vi "niFpgaDcRmsInsideSCTLWindow.vi"(0 "input data":fxp<+/-,32,1>, 1 "reset":bool, 9 "input valid":bool, 12 "ready for output":bool=TRUE) -> (2 "Sum result":fxp<+/-,42,11> format="%.35g", 4 "DC result":fxp<+/-,32,1> format="%.32g", 6 "RMS result":fxp<+,32,1> format="%.32g", 8 "Mean Square result":fxp<+,63,1> format="%.63g", 10 "results valid":bool, 14 "ready for input":bool)   [LabVIEW 2017]
uses:
  <vilib>/rvi/FXPMathLib/basic elements/FxpIntAccumulator/subVIs/nifxpmath_IntAccumulator_SimConfig.ctl
  <vilib>/rvi/FXPMathLib/basic elements/FxpIntAccumulator/simVIs/DllFxpIntAccumulator_sub.vi
  <vilib>/rvi/FXPMathLib/basic elements/FxpIntAccumulator/XNode/nifxpmath_IntAccumulator.xnode
  <vilib>/fxp/LVFixedPointOverflowPolicyTypeDef.ctl
  <vilib>/rvi/FXPMathLib/FxpMul/XNode/nifxpmath_Multiplier.xnode
  <vilib>/rvi/FXPMathLib/FxpSqrt/XNode/nifxpmath_Sqrt.xnode
  <vilib>/rvi/FXPMathLib/FxpSqrt/simVIs/DllSqrtTemp_sub.vi
  <vilib>/rvi/FXPMathLib/FxpSqrt/subVIs/nifxpmath_Sqrt_SimConfig.ctl
  <vilib>/rvi/FXPMathLib/sim/FxpSim.dll
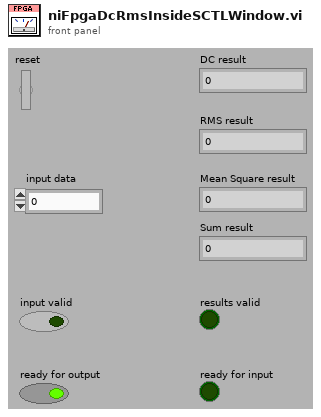
[diagram p1: front panel]
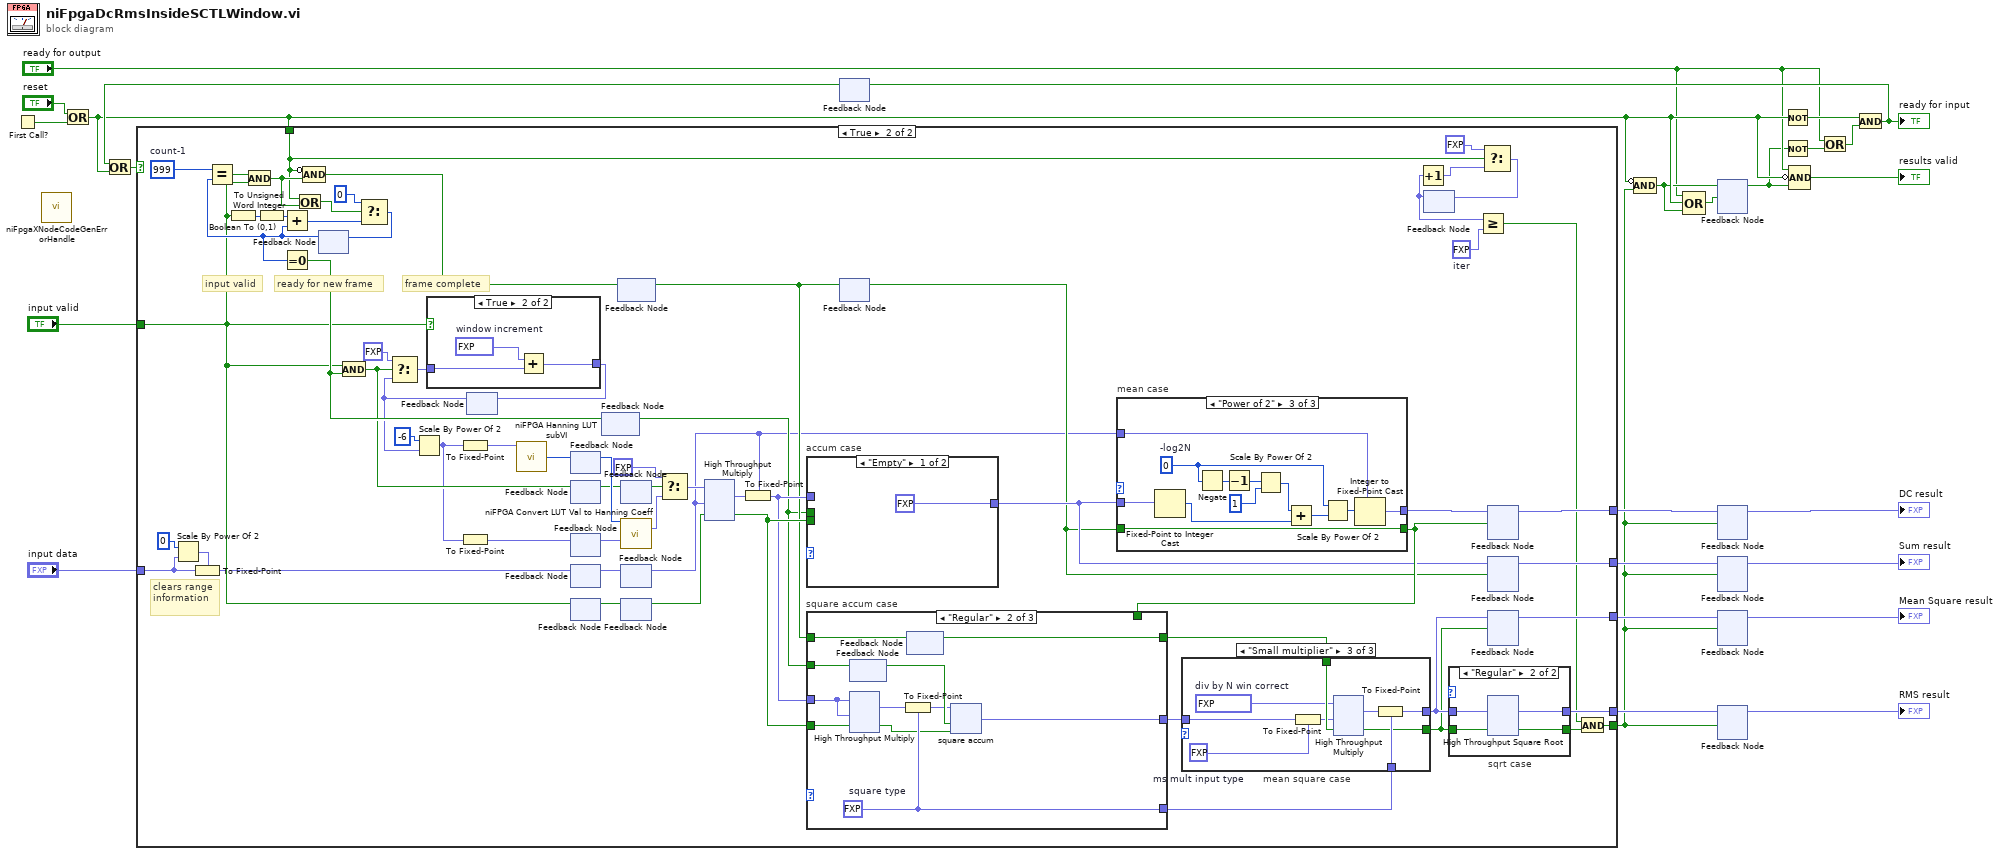
[diagram p0: block diagram]
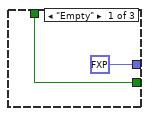
[diagram p4: hidden frame]
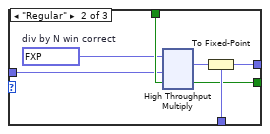
[diagram p5: hidden frame]
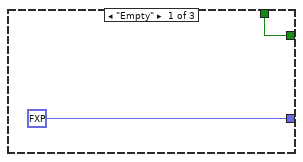
[diagram p6: hidden frame]
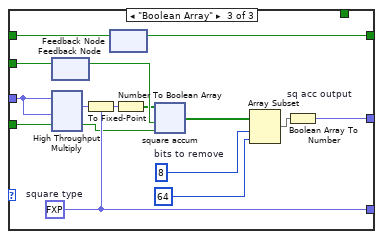
[diagram p7: hidden frame]
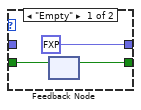
[diagram p8: hidden frame]
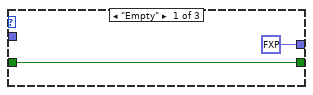
[diagram p9: hidden frame]
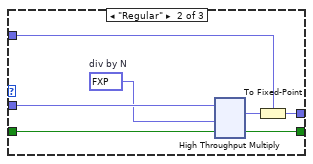
[diagram p10: hidden frame]
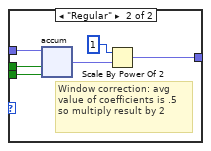
[diagram p11: hidden frame]
diagram:
  n1 = First Call?() -> (First Call?: T/F=w23:bool)
  n2 = call <vilib>:"niFpgaXNodeCodeGenErrorHandle.vi"() -> ()  [unwired: 1 in]
  n3 = Or(x="reset", y=w23) -> (x .or. y?=w6:bool)
  n4 = feedback #1() -> (w7:bool)  [unwired: 1 in]
  n5 = Or(x=w7, y=w6) -> (x .or. y?=w8:bool)
  n6 = case shown="True" w8 {
    tunnel: w6 -> [_ w78]
    tunnel: [_ w72] -> w16
    tunnel: [_ w71] -> w15
    tunnel: [_ w68] -> w14
    tunnel: [_ w66] -> w13
    tunnel: "input data" -> [_ w27]
    tunnel: "input valid" -> [_ w60]
    tunnel: [_ w52] -> w10
    frame False {
    }
    frame True {
      w80 = fxp<+,6,6> 43.0  # iter
      w76 = u16 999  # count-1
      # "clears range information"
      # "frame complete"
      # "ready for new frame"
      # "input valid"
      n7 = Scale By Power Of 2(n=0, x=w27) -> (x*2^n=w26:fxp<+/-,32,1>)
      n8 = To Fixed-Point(fixed-point type=w26, number=w27) -> (fixed-point=w42:fxp<+/-,32,1>)
      n9 = Boolean To (0,1)(Boolean=w60) -> (0, 1=w90:i16)
      n10 = To Unsigned Word Integer(number=w90) -> (unsigned 16bit integer=w75:u16)
      n11 = feedback #2() -> (w86:u16)  [unwired: 1 in]
      n12 = Equal?(x=w76, y=w86) -> (x = y?=w88:bool)
      n13 = And(x=w88, y=w60) -> (x .and. y?=w84:bool)
      n14 = Add(x=w75, y=w86) -> (x+y=w89:u16)
      n15 = Equal To 0?(x=w86) -> (x = 0?=w61:bool)
      n16 = Or(x=w78, y=w84) -> (x .or. y?=w85:bool)
      n17 = Compound Arithmetic op=AND(invert w78, w84) -> (w51:bool)
      n18 = And(x=w60, y=w61) -> (x .and. y?=w43:bool)
      n19 = Select(t=u16 0, s=w85, f=w89) -> (s? t:f=w77:u16)
      n20 = feedback-in #2(w77) -> ()
      n21 = feedback #3() -> (w39:fxp<+,32,16>)  [unwired: 1 in]
      n22 = Select(t=fxp<+,32,16> 0.0, s=w43, f=w39) -> (s? t:f=w62:fxp<+,32,16>)
      n23 = Scale By Power Of 2(n=-6, x=w39) -> (x*2^n=w38:fxp<+,32,16>)
      n24 = case shown="True" w60 {
        tunnel: [w91 w94] -> w63
        tunnel: w62 -> [w91 w92]
        frame False {
        }
        frame True {
          w93 = fxp<+,32,16> 65.53599548339844  # window increment
          n25 = Add(x=w93, y=w92) -> (x+y=w94:fxp<+,32,16>)
        }
      }
      n26 = To Fixed-Point(number=w38) -> (fixed-point=w30:fxp<+,10,10>)  [unwired: 1 in]
      n27 = To Fixed-Point(number=w38) -> (fixed-point=w40:fxp<+,16,0>)  [unwired: 1 in]
      n28 = feedback-in #3(w63) -> ()
      n29 = call <vilib>:"niFPGA Hanning LUT subVI.vi"("address"=w30) -> ("data out"=w29:u32)  [unwired: 7 in]
      n30 = feedback-in #4(w29) -> ()
      n31 = feedback #4() -> (w55:u32)  [unwired: 1 in]
      n32 = feedback-in #5(w43) -> ()
      n33 = feedback #5() -> (w32:bool)  [unwired: 1 in]
      n34 = feedback-in #6(w40) -> ()
      n35 = feedback #6() -> (w54:fxp<+,16,0>)  [unwired: 1 in]
      n36 = feedback-in #7(w42) -> ()
      n37 = feedback #7() -> (w36:fxp<+/-,32,1>)  [unwired: 1 in]
      n38 = feedback-in #8(w60) -> ()
      n39 = feedback #8() -> (w35:bool)  [unwired: 1 in]
      n40 = feedback-in #9(w61) -> ()
      n41 = feedback #9() -> (w48:bool)  [unwired: 1 in]
      n42 = feedback-in #10(w51) -> ()
      n43 = feedback #10() -> (w50:bool)  [unwired: 1 in]
      n44 = feedback-in #11(w32) -> ()
      n45 = feedback #11() -> (w31:bool)  [unwired: 1 in]
      n46 = call <vilib>:"niFPGA Convert LUT Val to Hanning Coeff.vi"("LUT value"=w55, "fractional index"=w54) -> ("Hanning coefficient"=w46:fxp<+,17,0>)  [unwired: 13 in]
      n47 = feedback-in #12(w36) -> ()
      n48 = feedback #12() -> (w33:fxp<+/-,32,1>)  [unwired: 1 in]
      n49 = feedback-in #13(w35) -> ()
      n50 = feedback #13() -> (w34:bool)  [unwired: 1 in]
      n51 = Select(t=fxp<+,17,0> 0.0, s=w31, f=w46) -> (s? t:f=w45:fxp<+,17,0>)
      n52 = xnode "High Throughput Multiply"("x"=w45, "y"=w33, "input valid"=w34) -> ("x*y"=w57:fxp<+/-,49,1>, "output valid"=w59:bool)  [unwired: 1 in, 1 out]
      n53 = To Fixed-Point(fixed-point type=w33, number=w57) -> (fixed-point=w56:fxp<+/-,32,1>)
      n54 = case "accum case" shown="\"Empty\"" {
        selector: _ -> [_ _]
        tunnel: w59 -> [_ w249]
        tunnel: w48 -> [_ w248]
        tunnel: w56 -> [_ w247]
        tunnel: [fxp<+/-,26,11> 0.0 ("s") w244] -> w58
        frame "Empty" {
        }
        frame "Regular" {
          # "Window correction: avg value of coefficients is .5 so multiply result by 2"
          n55 = xnode "accum"("x"=w247, "load (F)"=w248, "enable (T)"=w249) -> ("s"=w245:fxp<+/-,48,17>)  [unwired: 2 in, 1 out]
          n56 = Scale By Power Of 2(n=1, x=w245) -> (x*2^n=w244:fxp<+/-,48,17>)
        }
      }
      n57 = feedback-in #14(w50) -> ()
      n58 = feedback #14() -> (w49:bool)  [unwired: 1 in]
      n59 = case "mean case" shown="\"Power of 2\"" {
        selector: _ -> [_ _ _]
        tunnel: w33 -> [_ w230 w234]
        tunnel: w49 -> [w223 w229 w242]
        tunnel: w58 -> [_ w228 w232]
        tunnel: [w223 w227 w242] -> w65
        tunnel: [fxp<+/-,16,1> 0.0 ("input data") w226 w231] -> w67
        frame "Empty" {
        }
        frame "Regular" {
          w224 = fxp<+,17,-9> 0.0010000020265579224  # div by N
          n60 = xnode "High Throughput Multiply"("x"=w228, "y"=w224, "input valid"=w229) -> ("x*y"=w225:fxp<+/-,64,8>, "output valid"=w227:bool)  [unwired: 1 in, 1 out]
          n61 = To Fixed-Point(fixed-point type=w230, number=w225) -> (fixed-point=w226:fxp<+/-,32,1>)
        }
        frame "Power of 2" {
          w233 = i8 0  # -log2N
          n62 = Fixed-Point to Integer Cast(1:w232) -> (0:w237:i64)
          n63 = Negate(x=w233) -> (-x=w241:i8)
          n64 = Decrement(x=w241) -> (x-1=w240:i8)
          n65 = Scale By Power Of 2(n=w240, x=i64 1 ("x-1")) -> (x*2^n=w238:i64)
          n66 = Add(x=w238, y=w237) -> (x+y=w235:i64)
          n67 = Scale By Power Of 2(n=w233, x=w235) -> (x*2^n=w236:i64)
          n68 = Integer to Fixed-Point Cast(fixed-point type=w234, integer=w236) -> (fixed-point=w231:fxp<+/-,32,1>)
        }
      }
      n69 = case "square accum case" shown="\"Regular\"" {
        selector: _ -> [_ _ _]
        tunnel: w59 -> [_ w125 w168]
        tunnel: w48 -> [_ w124 w167]
        tunnel: w56 -> [_ w123 w166]
        tunnel: [_ w122 w165] -> w74
        tunnel: [w113 w117 w161] -> w70
        tunnel: [fxp<+,1,1> 0.0 ("s") w116 w153] -> w69
        tunnel: w50 -> [_ w115 w160]
        tunnel: w65 -> [w113 _ _]
        frame "Empty" {
        }
        frame "Regular" {
          w122 = fxp<+,63,1> 0.0  # square type
          n70 = feedback-in #15(w124) -> ()
          n71 = feedback #15() -> (w120:bool)  [unwired: 1 in]
          n72 = xnode "High Throughput Multiply"("x"=w123, "y"=w123, "input valid"=w125) -> ("x*y"=w119:fxp<+/-,64,2>, "output valid"=w121:bool)  [unwired: 1 in, 1 out]
          n73 = To Fixed-Point(fixed-point type=w122, number=w119) -> (fixed-point=w118:fxp<+,63,1>)
          n74 = feedback-in #16(w115) -> ()
          n75 = feedback #16() -> (w117:bool)  [unwired: 1 in]
          n76 = xnode "square accum"("x"=w118, "load (F)"=w120, "enable (T)"=w121) -> ("s"=w116:fxp<+,63,1>)  [unwired: 2 in, 1 out]
        }
        frame "Boolean Array" {
          w157 = 8  # bits to remove
          w165 = fxp<+,63,1> 0.0  # square type
          n77 = feedback-in #17(w167) -> ()
          n78 = feedback #17() -> (w163:bool)  [unwired: 1 in]
          n79 = xnode "High Throughput Multiply"("x"=w166, "y"=w166, "input valid"=w168) -> ("x*y"=w162:fxp<+/-,64,2>, "output valid"=w164:bool)  [unwired: 1 in, 1 out]
          n80 = To Fixed-Point(fixed-point type=w165, number=w162) -> (fixed-point=w159:fxp<+,63,1>)
          n81 = feedback-in #18(w160) -> ()
          n82 = feedback #18() -> (w161:bool)  [unwired: 1 in]
          n83 = Number To Boolean Array(number=w159) -> (Boolean array=w158:bool[])
          n84 = xnode "square accum"("x"=w158, "load (F)"=w163, "enable (T)"=w164) -> ("s"=w154:bool[])  [unwired: 2 in, 1 out]
          n85 = Array Subset(array=w154, index=w157, length=64) -> (w155:bool[])
          n86 = Boolean Array To Number "sq acc output"(Boolean array=w155) -> (number=w153:fxp<+,64,10>)
        }
      }
      n87 = case "mean square case" shown="\"Small multiplier\"" {
        selector: _ -> [_ _ _]
        tunnel: w74 -> [_ w103 w112]
        tunnel: [w96 w102 w111] -> w64
        tunnel: [fxp<+,1,1> 0.0 ("square type") w101 w110] -> w73
        tunnel: w70 -> [w96 w100 w109]
        tunnel: w69 -> [_ w99 w107]
        frame "Empty" {
        }
        frame "Regular" {
          w97 = fxp<+,17,-8> 0.0026667118072509766  # div by N win correct
          n88 = xnode ("High Throughput Multiply")("x"=w97, "y"=w99, "input valid"=w100) -> ("x*y"=w98:fxp<+,64,2>, "output valid"=w102:bool)  [unwired: 1 in, 1 out]
          n89 = To Fixed-Point(fixed-point type=w103, number=w98) -> (fixed-point=w101:fxp<+,63,1>)
        }
        frame "Small multiplier" {
          w104 = fxp<+,17,-8> 0.0026667118072509766  # div by N win correct
          w105 = fxp<+,34,10> 0.0  # ms mult input type
          n90 = To Fixed-Point(fixed-point type=w105, number=w107) -> (fixed-point=w106:fxp<+,34,10>)
          n91 = xnode ("High Throughput Multiply")("x"=w104, "y"=w106, "input valid"=w109) -> ("x*y"=w108:fxp<+,51,2>, "output valid"=w111:bool)  [unwired: 1 in, 1 out]
          n92 = To Fixed-Point(fixed-point type=w112, number=w108) -> (fixed-point=w110:fxp<+,63,1>)
        }
      }
      n93 = feedback #19() -> (w79:fxp<+,6,6>)  [unwired: 1 in]
      n94 = Increment(x=w79) -> (x+1=w82:fxp<+,6,6>)
      n95 = case "sqrt case" shown="\"Regular\"" {
        selector: _ -> [_ _]
        tunnel: [w191 w197] -> w53
        tunnel: w64 -> [w192 w196]
        tunnel: w73 -> [_ w195]
        tunnel: [fxp<+,1,1> 0.0 ("sqrt(x)") w194] -> w71
        frame "Empty" {
          n96 = feedback-in #20(w192) -> ()
          n97 = feedback #20() -> (w191:bool)  [unwired: 1 in]
        }
        frame "Regular" {
          n98 = xnode ("High Throughput Square Root")("x"=w195, "input valid"=w196) -> ("sqrt(x)"=w194:fxp<+,32,1>, "output valid"=w197:bool)  [unwired: 1 in, 1 out]
        }
      }
      n99 = Greater Or Equal?(x=w79, y=w80) -> (x >= y?=w47:bool)
      n100 = Select(t=fxp<+,1,1> 0.0, s=w78, f=w82) -> (s? t:f=w81:fxp<+,6,6>)
      n101 = feedback-in #19(w81) -> ()
      n102 = feedback-in #21(w67, w65) -> ()
      n103 = feedback #21() -> (w66:fxp<+/-,32,1>)  [unwired: 1 in]
      n104 = feedback-in #22(w58, w49) -> ()
      n105 = feedback #22() -> (w68:fxp<+/-,48,17>)  [unwired: 1 in]
      n106 = feedback-in #23(w73, w64) -> ()
      n107 = feedback #23() -> (w72:fxp<+,63,1>)  [unwired: 1 in]
      n108 = And(x=w47, y=w53) -> (x .and. y?=w52:bool)
    }
  }
  n109 = Compound Arithmetic op=AND(invert w6, w10) -> (w5:bool)
  n110 = Compound Arithmetic op=OR("ready for output", w6, w5) -> (w4:bool)
  n111 = feedback-in #24(w5, w4) -> ()
  n112 = feedback #24() -> (w1:bool)  [unwired: 1 in]
  n113 = feedback-in #25(w13, w10) -> ()
  n114 = feedback #25() -> (→"DC result":fxp<+/-,32,1>)  [unwired: 1 in]
  n115 = feedback-in #26(w14, w10) -> ()
  n116 = feedback #26() -> (→"Sum result":fxp<+/-,48,17>)  [unwired: 1 in]
  n117 = feedback-in #27(w16, w10) -> ()
  n118 = feedback #27() -> (→"Mean Square result":fxp<+,63,1>)  [unwired: 1 in]
  n119 = feedback-in #28(w15, w10) -> ()
  n120 = feedback #28() -> (→"RMS result":fxp<+,32,1>)  [unwired: 1 in]
  n121 = Not(x=w6) -> (.not. x?=w21:bool)
  n122 = Not(x=w1) -> (.not. x?=w2:bool)
  n123 = Compound Arithmetic op=AND("ready for output", invert w6, w1) -> (→"results valid":bool)
  n124 = Or(x="ready for output", y=w2) -> (x .or. y?=w20:bool)
  n125 = And(x=w21, y=w20) -> (x .and. y?=w9:bool)
  "ready for input" <- w9
  n126 = feedback-in #1(w9) -> ()
